vi "AB_1200_1300_Project_Build_Info.vi"(7 "action":T1, 8 "error in (no error)":errorcluster, 10 "buildInfo in":T2, 11 "Object In":T3) -> (0 "error out":errorcluster, 2 "buildInfo out":T2, 3 "Object Out":T3)   [LabVIEW 2020]
uses:
  <vilib>/AppBuilder/RW_Project/AB_RW_Project_PropBag_Action.ctl
  <resource>/Framework/Providers/API/ItemRef.ctl
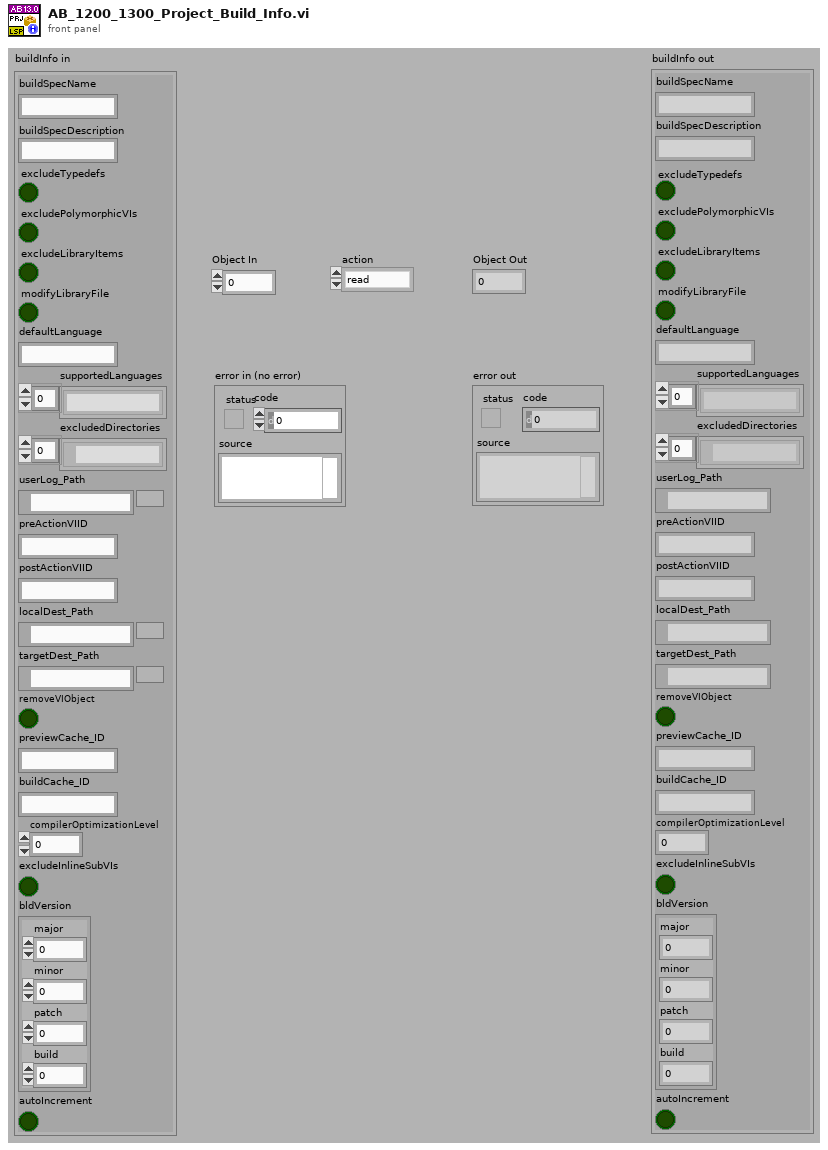
[diagram p1: front panel]
types:
  T1 = typedef "AB_RW_Project_PropBag_Action.ctl" = enum16{"read", "write", "clear", "readPrevious", "writePrevious", "clearPrevious"}
  T2 = cluster{"buildSpecName":string, "buildSpecDescription":string, "excludeTypedefs":bool, "excludePolymorphicVIs":bool, "excludeLibraryItems":bool, "modifyLibraryFile":bool, "defaultLanguage":string, "supportedLanguages":string[], "excludedDirectories":path[], "userLog_Path":path, "preActionVIID":string, "postActionVIID":string, "localDest_Path":path, "targetDest_Path":path, "removeVIObject":bool, "previewCache_ID":string, "buildCache_ID":string, "compilerOptimizationLevel":u32, "excludeInlineSubVIs":bool, "bldVersion":cluster{"major":u16, "minor":u16, "patch":u16, "build":u16}, "autoIncrement":bool}
  T3 = typedef "ItemRef.ctl" = u64
  T4 = cluster{"[0]":i32, "[1]":i32, "[2]":i32, "[3]":i32}
  T5 = cluster{"major":u16, "minor":u16, "patch":u16, "build":u16}
  T6 = typedef "AB_Relative_Path_Type.ctl" = enum16{"<none>", "relativeToCommon", "relativeToAppDir", "relativeToProject"}
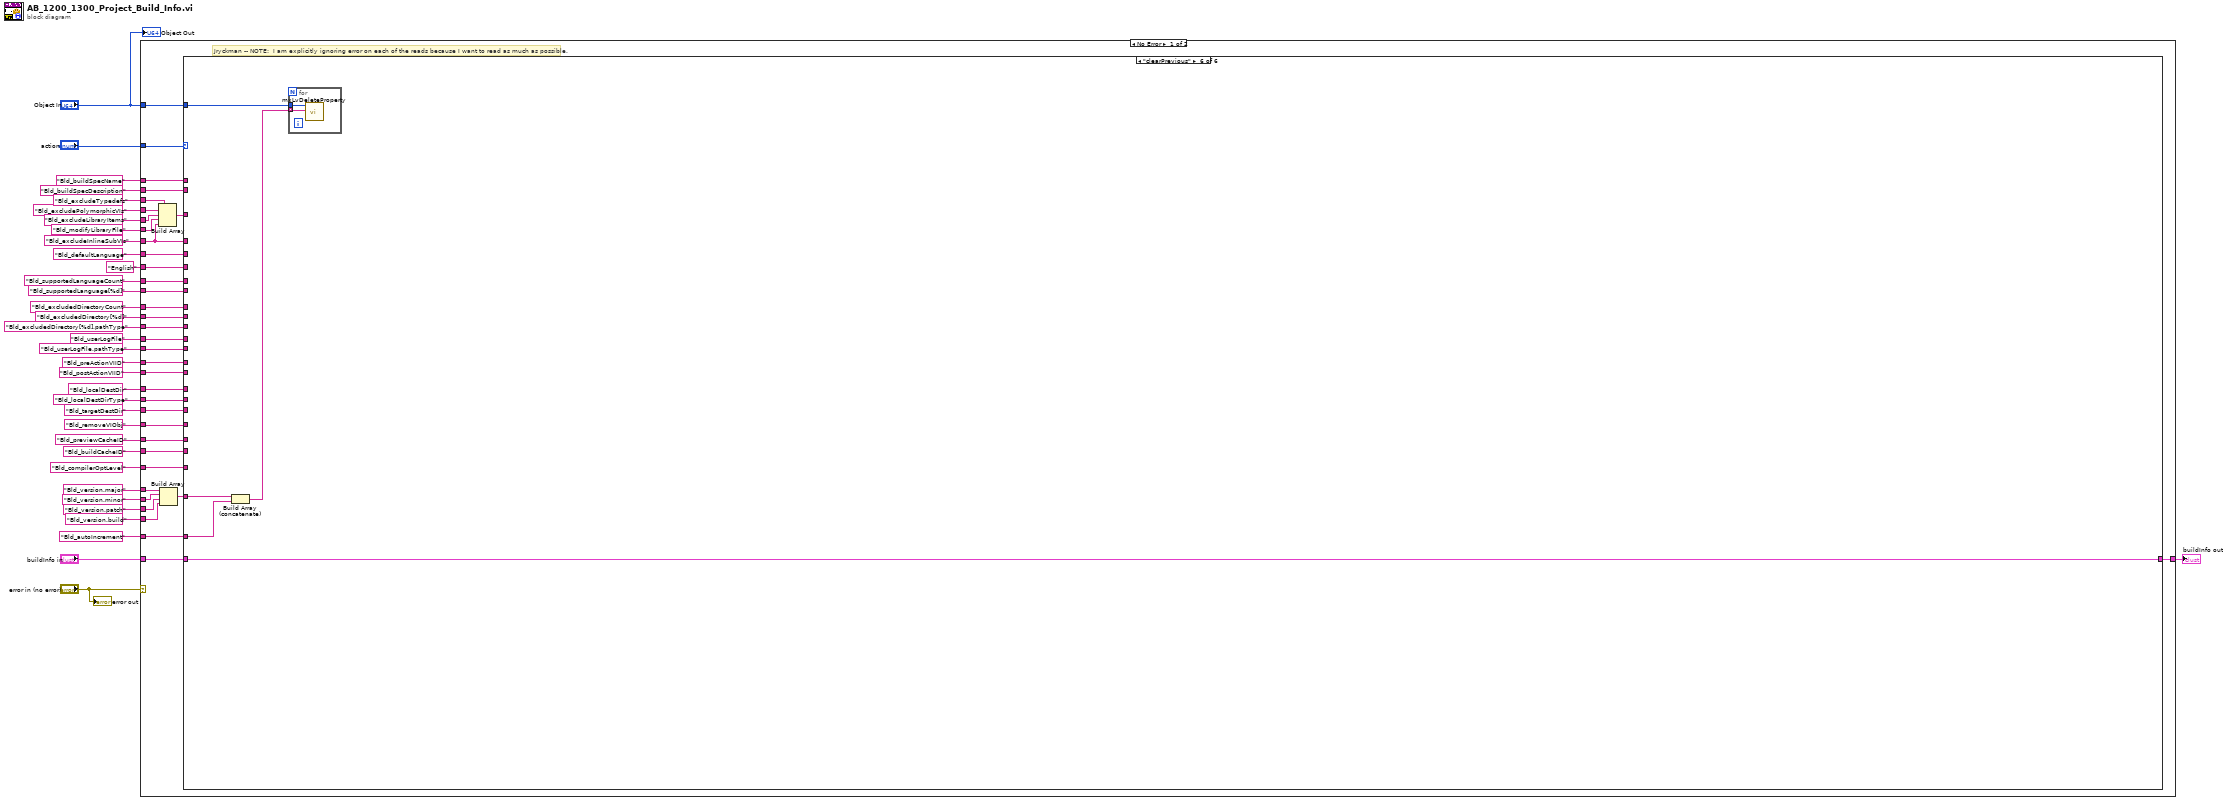
[diagram p0: block diagram]
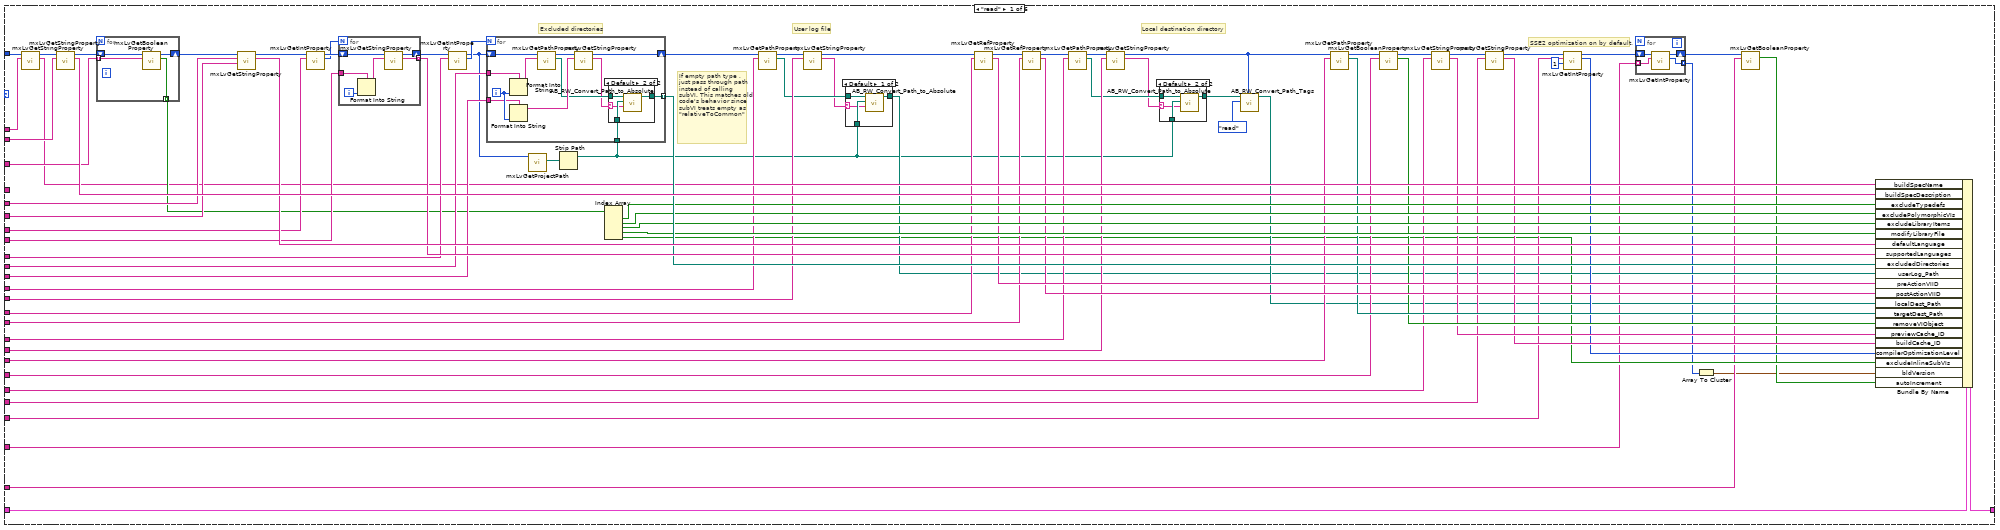
[diagram p2: hidden frame]
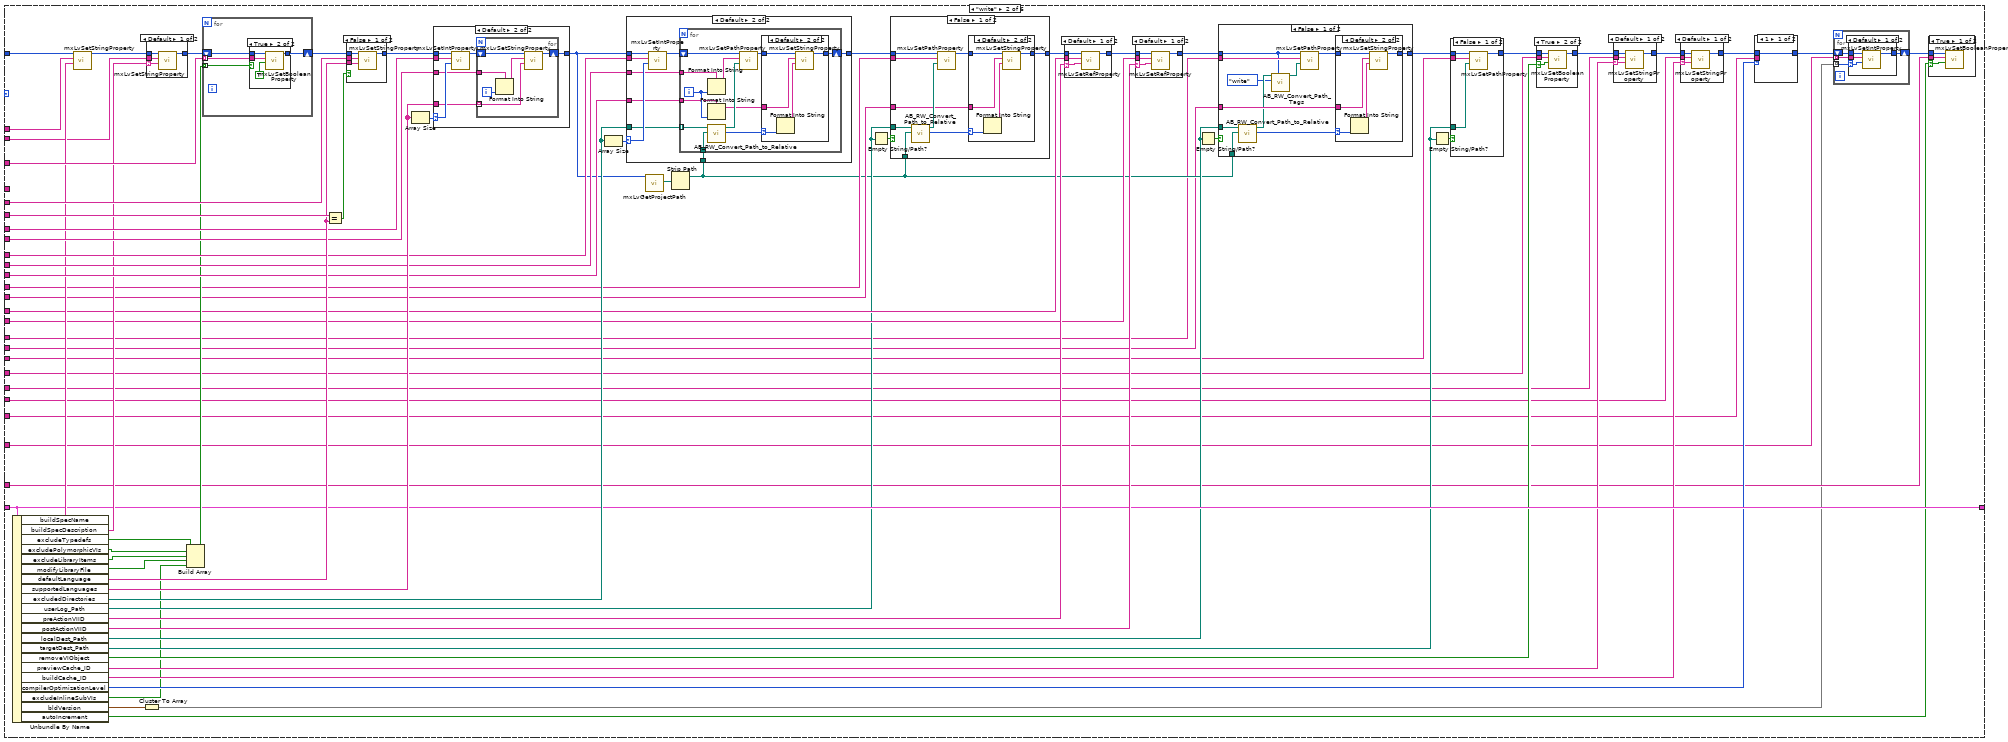
[diagram p6: hidden frame]
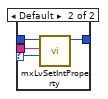
[diagram p9: hidden frame]
diagram:
  n1 = case shown="No Error" "error in (no error)" {
    tunnel: "Object In" -> [w71 _]
    tunnel: [w60 _] -> w33
    tunnel: "Bld_buildSpecDescription" ("Tag") -> [w70 _]
    tunnel: "Bld_excludeTypedefs" ("Tag") -> [w56 _]
    tunnel: "Bld_defaultLanguage" ("Tag") -> [w69 _]
    tunnel: "English" ("Tag") -> [w68 _]
    tunnel: "Bld_supportedLanguageCount" ("Tag") -> [w67 _]
    tunnel: "Bld_supportedLanguage[%d]" ("Tag") -> [w66 _]
    tunnel: "Bld_excludedDirectoryCount" ("Tag") -> [w65 _]
    tunnel: "Bld_excludedDirectory[%d]" ("Tag") -> [w64 _]
    tunnel: "Bld_excludedDirectory[%d].pathType" ("Tag") -> [w63 _]
    tunnel: "buildInfo in" -> [w62 _]
    tunnel: "action" -> [w61 _]
    tunnel: "Bld_excludePolymorphicVIs" ("Tag") -> [w59 _]
    tunnel: "Bld_excludeLibraryItems" ("Tag") -> [w58 _]
    tunnel: "Bld_modifyLibraryFile" ("Tag") -> [w57 _]
    tunnel: "Bld_buildSpecName" ("Tag") -> [w54 _]
    tunnel: "Bld_userLogFile" ("Tag") -> [w53 _]
    tunnel: "Bld_userLogFile.pathType" ("Tag") -> [w52 _]
    tunnel: "Bld_preActionVIID" ("Tag") -> [w51 _]
    tunnel: "Bld_postActionVIID" ("Tag") -> [w50 _]
    tunnel: "Bld_localDestDir" ("Tag") -> [w49 _]
    tunnel: "Bld_targetDestDir" ("Tag") -> [w48 _]
    tunnel: "Bld_localDestDirType" ("Tag") -> [w47 _]
    tunnel: "Bld_removeVIObj" ("Tag") -> [w46 _]
    tunnel: "Bld_previewCacheID" ("Tag") -> [w45 _]
    tunnel: "Bld_buildCacheID" ("Tag") -> [w44 _]
    tunnel: "Bld_compilerOptLevel" ("Tag") -> [w43 _]
    tunnel: "Bld_excludeInlineSubVIs" ("Tag") -> [w42 _]
    tunnel: "Bld_version.major" ("Tag") -> [w40 _]
    tunnel: "Bld_version.minor" ("Tag") -> [w39 _]
    tunnel: "Bld_version.patch" ("Tag") -> [w37 _]
    tunnel: "Bld_version.build" ("Tag") -> [w38 _]
    tunnel: "Bld_autoIncrement" ("Tag") -> [w41 _]
    frame No Error {
      # "Jryckman -- NOTE:  I am explicitly ignoring error on each of the reads because I want to read as much as possible."
      n2 = Build Array(w56, w59, w58, w57, w42) -> (w55:string[])
      n3 = Build Array(w40, w39, w37, w38) -> (w36:string[])
      n4 = case shown="\"clearPrevious\"" w61 {
        tunnel: w71 -> [w124 w243 w448 _ _ w474]
        tunnel: w70 -> [w151 w238 w450 _ _ _]
        tunnel: w69 -> [w149 w263 w449 _ _ _]
        tunnel: w68 -> [w148 w262 _ _ _ _]
        tunnel: w67 -> [w145 w257 w447 _ _ _]
        tunnel: w66 -> [w142 w256 w444 _ _ _]
        tunnel: w65 -> [w139 w252 w440 _ _ _]
        tunnel: w64 -> [w137 w251 w439 _ _ _]
        tunnel: w63 -> [w136 w250 w438 _ _ _]
        tunnel: w62 -> [w133 w222 w435 w470 w471 w476]
        tunnel: [w134 w222 w435 w470 w471 w476] -> w60
        tunnel: w55 -> [w130 w244 w434 _ _ _]
        tunnel: w54 -> [w122 w241 w433 _ _ _]
        tunnel: w53 -> [w117 w235 w431 _ _ _]
        tunnel: w52 -> [w115 w231 w429 _ _ _]
        tunnel: w51 -> [w114 w229 w426 _ _ _]
        tunnel: w50 -> [w111 w226 w425 _ _ _]
        tunnel: w49 -> [w106 w217 w422 _ _ _]
        tunnel: w48 -> [w104 w215 w420 _ _ _]
        tunnel: w47 -> [w105 w218 w421 _ _ _]
        tunnel: w46 -> [w100 w211 w417 _ _ _]
        tunnel: w45 -> [w98 w208 w415 _ _ _]
        tunnel: w44 -> [w95 w205 w413 _ _ _]
        tunnel: w43 -> [w91 w201 w411 _ _ _]
        tunnel: w42 -> [_ _ _ _ _ _]
        tunnel: w41 -> [w74 w196 w407 _ _ w472]
        tunnel: w36 -> [w76 w193 w409 _ _ w473]
        frame "read" {
          # "If empty path type , just pass through path instead of calling subVI. This matches old code's behavior since subVI treats empty as \"relativeToCommon\""
          # "Local destination directory"
          # "User log file"
          # "Excluded directories"
          # "SSE2 optimization on by default."
          n5 = call <resource>:"mxLvGetStringProperty.vi"("Tag"=w122, "Item"=w124) -> ("Value"=w121:string, "Item"=w123:T3)  [unwired: 1 in, 7 out]
          n6 = call <resource>:"mxLvGetStringProperty.vi"("Tag"=w151, "Item"=w123) -> ("Value"=w150:string, "Item"=w132:T3)  [unwired: 1 in, 7 out]
          n7 = for {
            shift-right: [w169] -> w131
            shift-left: w132 -> [w167]
            tunnel: w130 -> [w168] mode=indexing
            tunnel: [w166] -> w129 mode=indexing
            n8 = call <resource>:"mxLvGetBooleanProperty.vi"("Tag"=w168, "Item"=w167) -> ("Value"=w166:bool, "Item"=w169:T3)  [unwired: 1 in, 7 out]
          }
          n9 = call <resource>:"mxLvGetStringProperty.vi"("Default Value (\"\")"=w148, "Tag"=w149, "Item"=w131) -> ("Value"=w147:string, "Item"=w146:T3)  [unwired: 1 in, 6 out]
          n10 = call <resource>:"mxLvGetIntProperty.vi"("Tag"=w145, "Item"=w146) -> ("Value"=w143:i32, "Item"=w144:T3)  [unwired: 1 in, 7 out]
          n11 = for {
            N: w143 -> [_]
            shift-right: [w189] -> w140
            shift-left: w144 -> [w190]
            tunnel: w142 -> [w191]
            tunnel: [w187] -> w141 mode=indexing
            i -> [w192]
            n12 = Format Into String(format string=w191, w192) -> (resulting string=w188:string)  [unwired: 2 in, 1 out]
            n13 = call <resource>:"mxLvGetStringProperty.vi"("Tag"=w188, "Item"=w190) -> ("Value"=w187:string, "Item"=w189:T3)  [unwired: 1 in, 7 out]
          }
          n14 = call <resource>:"mxLvGetIntProperty.vi"("Tag"=w139, "Item"=w140) -> ("Value"=w138:i32, "Item"=w120:T3)  [unwired: 1 in, 7 out]
          n15 = call <resource>:"mxLvGetProjectPath.vi"("Item"=w120) -> ("Project Path"=w119:path)  [unwired: 1 in, 9 out]
          n16 = Strip Path(path=w119) -> (stripped path=w82:path)  [unwired: 1 out]
          n17 = for {
            N: w138 -> [_]
            shift-right: [w174] -> w118
            shift-left: w120 -> [w178]
            tunnel: w137 -> [w181]
            tunnel: w136 -> [w179]
            tunnel: w82 -> [w171]
            tunnel: [w172] -> w135 mode=indexing
            i -> [w180]
            n18 = Format Into String(format string=w181, w180) -> (resulting string=w177:string)  [unwired: 2 in, 1 out]
            n19 = Format Into String(format string=w179, w180) -> (resulting string=w175:string)  [unwired: 2 in, 1 out]
            n20 = call <resource>:"mxLvGetPathProperty.vi"("Tag"=w177, "Item"=w178) -> ("Path"=w173:path, "Item"=w176:T3)  [unwired: 2 in, 6 out]
            n21 = call <resource>:"mxLvGetStringProperty.vi"("Tag"=w175, "Item"=w176) -> ("Value"=w170:string, "Item"=w174:T3)  [unwired: 1 in, 7 out]
            n22 = case shown="Default" w170 {
              selector: w170 -> [_ w183]
              tunnel: w173 -> [w182 w186]
              tunnel: [w182 w185] -> w172
              tunnel: w171 -> [_ w184]
              frame "" {
              }
              frame Default {
                n23 = call <vilib>:"AB_RW_Convert_Path_to_Absolute.vi"("relativeType"=w183, "commonPath"=w184, "relativePath"=w186) -> ("absolute path"=w185:path)  [unwired: 7 in, 1 out]
              }
            }
          }
          n24 = Index Array(array=w129) -> (element #1=w128:bool, element #2=w127:bool, element #3=w126:bool, element #4=w125:bool, element #5=w79:bool)  [unwired: 5 in]
          n25 = call <resource>:"mxLvGetPathProperty.vi"("Tag"=w117, "Item"=w118) -> ("Path"=w86:path, "Item"=w116:T3)  [unwired: 2 in, 6 out]
          n26 = call <resource>:"mxLvGetStringProperty.vi"("Tag"=w115, "Item"=w116) -> ("Value"=w81:string, "Item"=w113:T3)  [unwired: 1 in, 7 out]
          n27 = case shown="Default" w81 {
            selector: w81 -> [w161 _]
            tunnel: w86 -> [w164 w165]
            tunnel: [w163 w165] -> w85
            tunnel: w82 -> [w162 _]
            frame Default {
              n28 = call <vilib>:"AB_RW_Convert_Path_to_Absolute.vi"("relativeType"=w161, "commonPath"=w162, "relativePath"=w164) -> ("absolute path"=w163:path)  [unwired: 7 in, 1 out]
            }
            frame "" {
            }
          }
          n29 = call <resource>:"mxLvGetRefProperty.vi"("Tag"=w114, "Item"=w113) -> ("Value"=w112:string, "Item"=w110:T3)  [unwired: 1 in, 7 out]
          n30 = call <resource>:"mxLvGetRefProperty.vi"("Tag"=w111, "Item"=w110) -> ("Value"=w109:string, "Item"=w107:T3)  [unwired: 1 in, 7 out]
          n31 = call <resource>:"mxLvGetPathProperty.vi"("Tag"=w106, "Item"=w107) -> ("Path"=w84:path, "Item"=w108:T3)  [unwired: 2 in, 6 out]
          n32 = call <resource>:"mxLvGetStringProperty.vi"("Tag"=w105, "Item"=w108) -> ("Value"=w80:string, "Item"=w88:T3)  [unwired: 1 in, 7 out]
          n33 = case shown="Default" w80 {
            selector: w80 -> [_ w157]
            tunnel: w84 -> [w156 w160]
            tunnel: [w156 w159] -> w83
            tunnel: w82 -> [_ w158]
            frame "" {
            }
            frame Default {
              n34 = call <vilib>:"AB_RW_Convert_Path_to_Absolute.vi"("relativeType"=w157, "commonPath"=w158, "relativePath"=w160) -> ("absolute path"=w159:path)  [unwired: 7 in, 1 out]
            }
          }
          n35 = call <vilib>:"AB_RW_Convert_Path_Tags.vi"("buildObject"=w88, "action"=AB_RW_Project_PropBag_Action."read", "Path in"=w83) -> ("Path out"=w89:path)  [unwired: 1 in, 7 out]
          n36 = call <resource>:"mxLvGetPathProperty.vi"("Tag"=w104, "Item"=w88) -> ("Path"=w103:path, "Item"=w102:T3)  [unwired: 2 in, 6 out]
          n37 = call <resource>:"mxLvGetBooleanProperty.vi"("Tag"=w100, "Item"=w102) -> ("Value"=w101:bool, "Item"=w99:T3)  [unwired: 1 in, 7 out]
          n38 = call <resource>:"mxLvGetStringProperty.vi"("Tag"=w98, "Item"=w99) -> ("Value"=w97:string, "Item"=w96:T3)  [unwired: 1 in, 7 out]
          n39 = call <resource>:"mxLvGetStringProperty.vi"("Tag"=w95, "Item"=w96) -> ("Value"=w94:string, "Item"=w93:T3)  [unwired: 1 in, 7 out]
          n40 = call <resource>:"mxLvGetIntProperty.vi"("Default Value (0)"=1, "Tag"=w91, "Item"=w93) -> ("Value"=w92:i32, "Item"=w77:T3)  [unwired: 1 in, 6 out]
          n41 = for {
            shift-right: [w154] -> w75
            shift-left: w77 -> [w155]
            tunnel: w76 -> [w152] mode=indexing
            tunnel: [w153] -> w78 mode=indexing
            n42 = call <resource>:"mxLvGetIntProperty.vi"("Tag"=w152, "Item"=w155) -> ("Value"=w153:i32, "Item"=w154:T3)  [unwired: 1 in, 7 out]
          }
          n43 = Array To Cluster(array=w78) -> (cluster=w72:T4)
          n44 = call <resource>:"mxLvGetBooleanProperty.vi"("Tag"=w74, "Item"=w75) -> ("Value"=w73:bool)  [unwired: 1 in, 8 out]
          n45 = Bundle By Name(cluster=w133, "buildSpecName"=w121, "buildSpecDescription"=w150, "excludeTypedefs"=w128, "excludePolymorphicVIs"=w127, "excludeLibraryItems"=w126, "modifyLibraryFile"=w125, "defaultLanguage"=w147, "supportedLanguages"=w141, "excludedDirectories"=w135, "userLog_Path"=w85, "preActionVIID"=w112, "postActionVIID"=w109, "localDest_Path"=w89, "targetDest_Path"=w103, "removeVIObject"=w101, "previewCache_ID"=w97, "buildCache_ID"=w94, "compilerOptimizationLevel"=w92, "excludeInlineSubVIs"=w79, "bldVersion"=w72, "autoIncrement"=w73) -> (w134:T2)
        }
        frame "write" {
          n46 = Unbundle By Name(w222) -> ("buildSpecName"=w242:string, "buildSpecDescription"=w237:string, "excludeTypedefs"=w249:bool, "excludePolymorphicVIs"=w248:bool, "excludeLibraryItems"=w247:bool, "modifyLibraryFile"=w246:bool, "defaultLanguage"=w261:string, "supportedLanguages"=w255:string[], "excludedDirectories"=w253:path[], "userLog_Path"=w221:path, "preActionVIID"=w228:string, "postActionVIID"=w225:string, "localDest_Path"=w220:path, "targetDest_Path"=w214:path, "removeVIObject"=w210:bool, "previewCache_ID"=w207:string, "buildCache_ID"=w204:string, "compilerOptimizationLevel"=w202:u32, "excludeInlineSubVIs"=w200:bool, "bldVersion"=w195:T5, "autoIncrement"=w197:bool)
          n47 = call <resource>:"mxLvSetStringProperty.vi"("Value (\"\")"=w242, "Tag"=w241, "Item"=w243) -> ("Item"=w240:T3)  [unwired: 2 in, 6 out]
          n48 = Cluster To Array(cluster=w195) -> (array=w194:u16[])
          n49 = case shown="Default" w237 {
            selector: w237 -> [w346 _]
            tunnel: w240 -> [w349 w350]
            tunnel: w238 -> [w348 _]
            tunnel: [w347 w350] -> w239
            frame Default {
              n50 = call <resource>:"mxLvSetStringProperty.vi"("Value (\"\")"=w346, "Tag"=w348, "Item"=w349) -> ("Item"=w347:T3)  [unwired: 2 in, 6 out]
            }
            frame "" {
            }
          }
          n51 = Build Array(w249, w248, w247, w246, w200) -> (w245:bool[])
          n52 = for {
            shift-right: [w353] -> w264
            shift-left: w239 -> [w354]
            tunnel: w245 -> [w352] mode=indexing
            tunnel: w244 -> [w351] mode=indexing
            n53 = case shown="True" w352 {
              tunnel: w354 -> [w355 w359]
              tunnel: [w355 w358] -> w353
              tunnel: w351 -> [_ w357]
              frame False {
              }
              frame True {
                n54 = call <resource>:"mxLvSetBooleanProperty.vi"("Value (F)"=TRUE, "Tag"=w357, "Item"=w359) -> ("Item"=w358:T3)  [unwired: 2 in, 6 out]
              }
            }
          }
          n55 = Equal?(x=w262, y=w261) -> (x = y?=w260:bool)
          n56 = case shown="False" w260 {
            tunnel: w264 -> [w405 w406]
            tunnel: w263 -> [w404 _]
            tunnel: w261 -> [w403 _]
            tunnel: [w402 w406] -> w258
            frame False {
              n57 = call <resource>:"mxLvSetStringProperty.vi"("Value (\"\")"=w403, "Tag"=w404, "Item"=w405) -> ("Item"=w402:T3)  [unwired: 2 in, 6 out]
            }
            frame True {
            }
          }
          n58 = Array Size(array=w255) -> (size(s)=w259:i32)
          n59 = case shown="Default" w259 {
            selector: w259 -> [_ w393]
            tunnel: w258 -> [w388 w395]
            tunnel: w257 -> [_ w394]
            tunnel: w256 -> [_ w391]
            tunnel: w255 -> [_ w390]
            tunnel: [w388 w389] -> w232
            frame 0 {
            }
            frame Default {
              n60 = call <resource>:"mxLvSetIntProperty.vi"("Value (0)"=w393, "Tag"=w394, "Item"=w395) -> ("Item"=w392:T3)  [unwired: 2 in, 6 out]
              n61 = for {
                shift-right: [w400] -> w389
                shift-left: w392 -> [w401]
                tunnel: w391 -> [w398]
                tunnel: w390 -> [w396] mode=indexing
                i -> [w399]
                n62 = Format Into String(format string=w398, w399) -> (resulting string=w397:string)  [unwired: 2 in, 1 out]
                n63 = call <resource>:"mxLvSetStringProperty.vi"("Value (\"\")"=w396, "Tag"=w397, "Item"=w401) -> ("Item"=w400:T3)  [unwired: 2 in, 6 out]
              }
            }
          }
          n64 = Array Size(array=w253) -> (size(s)=w254:i32)
          n65 = call <resource>:"mxLvGetProjectPath.vi"("Item"=w232) -> ("Project Path"=w233:path)  [unwired: 1 in, 9 out]
          n66 = Strip Path(path=w233) -> (stripped path=w219:path)  [unwired: 1 out]
          n67 = case shown="Default" w254 {
            selector: w254 -> [_ w368]
            tunnel: w232 -> [w360 w363]
            tunnel: w252 -> [_ w369]
            tunnel: w251 -> [_ w366]
            tunnel: w253 -> [_ w365]
            tunnel: w250 -> [_ w364]
            tunnel: [w360 w362] -> w236
            tunnel: w219 -> [_ w361]
            frame 0 {
            }
            frame Default {
              n68 = call <resource>:"mxLvSetIntProperty.vi"("Value (0)"=w368, "Tag"=w369, "Item"=w363) -> ("Item"=w367:T3)  [unwired: 2 in, 6 out]
              n69 = for {
                shift-right: [w381] -> w362
                shift-left: w367 -> [w377]
                tunnel: w366 -> [w380]
                tunnel: w365 -> [w379] mode=indexing
                tunnel: w361 -> [w371]
                tunnel: w364 -> [w370]
                i -> [w375]
                n70 = Format Into String(format string=w380, w375) -> (resulting string=w378:string)  [unwired: 2 in, 1 out]
                n71 = Format Into String(format string=w370, w375) -> (resulting string=w373:string)  [unwired: 2 in, 1 out]
                n72 = call <vilib>:"AB_RW_Convert_Path_to_Relative.vi"("commonPath"=w371, "absolutePath"=w379) -> ("relativeType"=w372:T6, "newPath"=w374:path)  [unwired: 1 in, 7 out]
                n73 = call <resource>:"mxLvSetPathProperty.vi"("Path"=w374, "Tag"=w378, "Item"=w377) -> ("Item"=w376:T3)  [unwired: 2 in, 6 out]
                n74 = case shown="Default" w372 {
                  selector: w372 -> [_ w383]
                  tunnel: [w382 w387] -> w381
                  tunnel: w376 -> [w382 w386]
                  tunnel: w373 -> [_ w384]
                  frame "<none>" {
                  }
                  frame Default {
                    n75 = Format Into String(w383) -> (resulting string=w385:string)  [unwired: 3 in, 1 out]
                    n76 = call <resource>:"mxLvSetStringProperty.vi"("Value (\"\")"=w385, "Tag"=w384, "Item"=w386) -> ("Item"=w387:T3)  [unwired: 2 in, 6 out]
                  }
                }
              }
            }
          }
          n77 = Empty String/Path?(string/path=w221) -> (empty?=w234:bool)
          n78 = case shown="False" w234 {
            tunnel: w236 -> [w338 w345]
            tunnel: w235 -> [w337 _]
            tunnel: w219 -> [w334 _]
            tunnel: w221 -> [w333 _]
            tunnel: w231 -> [w331 _]
            tunnel: [w330 w345] -> w230
            frame False {
              n79 = call <vilib>:"AB_RW_Convert_Path_to_Relative.vi"("commonPath"=w334, "absolutePath"=w333) -> ("relativeType"=w336:T6, "newPath"=w332:path)  [unwired: 1 in, 7 out]
              n80 = call <resource>:"mxLvSetPathProperty.vi"("Path"=w332, "Tag"=w337, "Item"=w338) -> ("Item"=w335:T3)  [unwired: 2 in, 6 out]
              n81 = case shown="Default" w336 {
                selector: w336 -> [_ w341]
                tunnel: w335 -> [w339 w344]
                tunnel: w331 -> [_ w342]
                tunnel: [w339 w340] -> w330
                frame "<none>" {
                }
                frame Default {
                  n82 = Format Into String(w341) -> (resulting string=w343:string)  [unwired: 3 in, 1 out]
                  n83 = call <resource>:"mxLvSetStringProperty.vi"("Value (\"\")"=w343, "Tag"=w342, "Item"=w344) -> ("Item"=w340:T3)  [unwired: 2 in, 6 out]
                }
              }
            }
            frame True {
            }
          }
          n84 = case shown="Default" w228 {
            selector: w228 -> [w326 _]
            tunnel: w230 -> [w328 w329]
            tunnel: w229 -> [w327 _]
            tunnel: [w325 w329] -> w227
            frame Default {
              n85 = call <resource>:"mxLvSetRefProperty.vi"("Value (\"\")"=w326, "Tag"=w327, "Item"=w328) -> ("Item"=w325:T3)  [unwired: 2 in, 6 out]
            }
            frame "" {
            }
          }
          n86 = case shown="Default" w225 {
            selector: w225 -> [w321 _]
            tunnel: w227 -> [w323 w324]
            tunnel: w226 -> [w322 _]
            tunnel: [w320 w324] -> w223
            frame Default {
              n87 = call <resource>:"mxLvSetRefProperty.vi"("Value (\"\")"=w321, "Tag"=w322, "Item"=w323) -> ("Item"=w320:T3)  [unwired: 2 in, 6 out]
            }
            frame "" {
            }
          }
          n88 = Empty String/Path?(string/path=w220) -> (empty?=w224:bool)
          n89 = case shown="False" w224 {
            tunnel: w223 -> [w302 w319]
            tunnel: w217 -> [w312 _]
            tunnel: w219 -> [w309 _]
            tunnel: w220 -> [w308 _]
            tunnel: w218 -> [w307 _]
            tunnel: [w306 w319] -> w216
            frame False {
              n90 = call <vilib>:"AB_RW_Convert_Path_to_Relative.vi"("commonPath"=w309, "absolutePath"=w308) -> ("relativeType"=w311:T6, "newPath"=w305:path)  [unwired: 1 in, 7 out]
              n91 = call <vilib>:"AB_RW_Convert_Path_Tags.vi"("buildObject"=w302, "action"=AB_RW_Project_PropBag_Action."write", "Path in"=w305) -> ("Path out"=w304:path)  [unwired: 1 in, 7 out]
              n92 = call <resource>:"mxLvSetPathProperty.vi"("Path"=w304, "Tag"=w312, "Item"=w302) -> ("Item"=w310:T3)  [unwired: 2 in, 6 out]
              n93 = case shown="Default" w311 {
                selector: w311 -> [_ w315]
                tunnel: w310 -> [w313 w318]
                tunnel: w307 -> [_ w316]
                tunnel: [w313 w314] -> w306
                frame "<none>" {
                }
                frame Default {
                  n94 = Format Into String(w315) -> (resulting string=w317:string)  [unwired: 3 in, 1 out]
                  n95 = call <resource>:"mxLvSetStringProperty.vi"("Value (\"\")"=w317, "Tag"=w316, "Item"=w318) -> ("Item"=w314:T3)  [unwired: 2 in, 6 out]
                }
              }
            }
            frame True {
            }
          }
          n96 = Empty String/Path?(string/path=w214) -> (empty?=w213:bool)
          n97 = case shown="False" w213 {
            tunnel: w216 -> [w300 w301]
            tunnel: w215 -> [w299 _]
            tunnel: w214 -> [w298 _]
            tunnel: [w297 w301] -> w212
            frame False {
              n98 = call <resource>:"mxLvSetPathProperty.vi"("Path"=w298, "Tag"=w299, "Item"=w300) -> ("Item"=w297:T3)  [unwired: 2 in, 6 out]
            }
            frame True {
            }
          }
          n99 = case shown="True" w210 {
            selector: w210 -> [_ w294]
            tunnel: w212 -> [w292 w296]
            tunnel: w211 -> [_ w295]
            tunnel: [w292 w293] -> w209
            frame False {
            }
            frame True {
              n100 = call <resource>:"mxLvSetBooleanProperty.vi"("Value (F)"=w294, "Tag"=w295, "Item"=w296) -> ("Item"=w293:T3)  [unwired: 2 in, 6 out]
            }
          }
          n101 = case shown="Default" w207 {
            selector: w207 -> [w288 _]
            tunnel: w209 -> [w290 w291]
            tunnel: w208 -> [w289 _]
            tunnel: [w287 w291] -> w206
            frame Default {
              n102 = call <resource>:"mxLvSetStringProperty.vi"("Value (\"\")"=w288, "Tag"=w289, "Item"=w290) -> ("Item"=w287:T3)  [unwired: 2 in, 6 out]
            }
            frame "" {
            }
          }
          n103 = case shown="Default" w204 {
            selector: w204 -> [w283 _]
            tunnel: w206 -> [w285 w286]
            tunnel: w205 -> [w284 _]
            tunnel: [w282 w286] -> w203
            frame Default {
              n104 = call <resource>:"mxLvSetStringProperty.vi"("Value (\"\")"=w283, "Tag"=w284, "Item"=w285) -> ("Item"=w282:T3)  [unwired: 2 in, 6 out]
            }
            frame "" {
            }
          }
          n105 = case shown="1" w202 {
            selector: w202 -> [_ w280]
            tunnel: w203 -> [w277 w281]
            tunnel: w201 -> [_ w279]
            tunnel: [w277 w278] -> w199
            frame 1 {
            }
            frame Default {
              n106 = call <resource>:"mxLvSetIntProperty.vi"("Value (0)"=w280, "Tag"=w279, "Item"=w281) -> ("Item"=w278:T3)  [unwired: 2 in, 6 out]
            }
          }
          n107 = for {
            tunnel: w194 -> [w270] mode=indexing
            shift-right: [w269] -> w198
            shift-left: w199 -> [w271]
            tunnel: w193 -> [w268] mode=indexing
            n108 = case shown="Default" w270 {
              selector: w270 -> [w274 _]
              tunnel: w271 -> [w275 w276]
              tunnel: w268 -> [w273 _]
              tunnel: [w272 w276] -> w269
              frame Default {
                n109 = call <resource>:"mxLvSetIntProperty.vi"("Value (0)"=w274, "Tag"=w273, "Item"=w275) -> ("Item"=w272:T3)  [unwired: 2 in, 6 out]
              }
              frame 0 {
              }
            }
          }
          n110 = case shown="True" w197 {
            selector: w197 -> [w266 _]
            tunnel: w198 -> [w267 _]
            tunnel: w196 -> [w265 _]
            frame True {
              n111 = call <resource>:"mxLvSetBooleanProperty.vi"("Value (F)"=w266, "Tag"=w265, "Item"=w267) -> ()  [unwired: 2 in, 7 out]
            }
            frame False {
            }
          }
        }
        frame "clear" {
          n112 = Build Array (concatenate)(w433, w450, w434, w449, w447, w440) -> (w436:string[])
          n113 = call <resource>:"mxLvGetIntProperty.vi"("Tag"=w447, "Item"=w448) -> ("Value"=w445:i32, "Item"=w446:T3)  [unwired: 1 in, 7 out]
          n114 = for {
            N: w445 -> [_]
            shift-right: [w466] -> w441
            shift-left: w446 -> [w467]
            tunnel: w444 -> [w468]
            i -> [w469]
            n115 = Format Into String(format string=w468, w469) -> (resulting string=w465:string)  [unwired: 2 in, 1 out]
            n116 = call <resource>:"mxLvDeleteProperty.vi"("Tag"=w465, "Item"=w467) -> ("Item"=w466:T3)  [unwired: 1 in, 8 out]
          }
          n117 = call <resource>:"mxLvGetIntProperty.vi"("Tag"=w440, "Item"=w441) -> ("Value"=w443:i32, "Item"=w442:T3)  [unwired: 1 in, 7 out]
          n118 = for {
            N: w443 -> [_]
            shift-right: [w460] -> w437
            shift-left: w442 -> [w463]
            tunnel: w439 -> [w464]
            tunnel: w438 -> [w458]
            i -> [w459]
            n119 = Format Into String(format string=w464, w459) -> (resulting string=w462:string)  [unwired: 2 in, 1 out]
            n120 = Format Into String(format string=w458, w459) -> (resulting string=w457:string)  [unwired: 2 in, 1 out]
            n121 = call <resource>:"mxLvDeleteProperty.vi"("Tag"=w462, "Item"=w463) -> ("Item"=w461:T3)  [unwired: 1 in, 8 out]
            n122 = call <resource>:"mxLvDeleteProperty.vi"("Tag"=w457, "Item"=w461) -> ("Item"=w460:T3)  [unwired: 1 in, 8 out]
          }
          n123 = for {
            tunnel: w436 -> [w455] mode=indexing
            shift-right: [w454] -> w432
            shift-left: w437 -> [w456]
            n124 = call <resource>:"mxLvDeleteProperty.vi"("Tag"=w455, "Item"=w456) -> ("Item"=w454:T3)  [unwired: 1 in, 8 out]
          }
          n125 = call <resource>:"mxLvDeleteProperty.vi"("Tag"=w431, "Item"=w432) -> ("Item"=w430:T3)  [unwired: 1 in, 8 out]
          n126 = call <resource>:"mxLvDeleteProperty.vi"("Tag"=w429, "Item"=w430) -> ("Item"=w427:T3)  [unwired: 1 in, 8 out]
          n127 = call <resource>:"mxLvDeleteProperty.vi"("Tag"=w426, "Item"=w427) -> ("Item"=w428:T3)  [unwired: 1 in, 8 out]
          n128 = call <resource>:"mxLvDeleteProperty.vi"("Tag"=w425, "Item"=w428) -> ("Item"=w419:T3)  [unwired: 1 in, 8 out]
          n129 = call <resource>:"mxLvDeleteProperty.vi"("Tag"=w422, "Item"=w419) -> ("Item"=w424:T3)  [unwired: 1 in, 8 out]
          n130 = call <resource>:"mxLvDeleteProperty.vi"("Tag"=w421, "Item"=w424) -> ("Item"=w423:T3)  [unwired: 1 in, 8 out]
          n131 = call <resource>:"mxLvDeleteProperty.vi"("Tag"=w420, "Item"=w423) -> ("Item"=w418:T3)  [unwired: 1 in, 8 out]
          n132 = call <resource>:"mxLvDeleteProperty.vi"("Tag"=w417, "Item"=w418) -> ("Item"=w416:T3)  [unwired: 1 in, 8 out]
          n133 = call <resource>:"mxLvDeleteProperty.vi"("Tag"=w415, "Item"=w416) -> ("Item"=w414:T3)  [unwired: 1 in, 8 out]
          n134 = call <resource>:"mxLvDeleteProperty.vi"("Tag"=w413, "Item"=w414) -> ("Item"=w412:T3)  [unwired: 1 in, 8 out]
          n135 = call <resource>:"mxLvDeleteProperty.vi"("Tag"=w411, "Item"=w412) -> ("Item"=w410:T3)  [unwired: 1 in, 8 out]
          n136 = for {
            tunnel: w409 -> [w452] mode=indexing
            shift-right: [w451] -> w408
            shift-left: w410 -> [w453]
            n137 = call <resource>:"mxLvDeleteProperty.vi"("Tag"=w452, "Item"=w453) -> ("Item"=w451:T3)  [unwired: 1 in, 8 out]
          }
          n138 = call <resource>:"mxLvDeleteProperty.vi"("Tag"=w407, "Item"=w408) -> ()  [unwired: 1 in, 9 out]
        }
        frame "readPrevious" {
        }
        frame "writePrevious" {
        }
        frame "clearPrevious" {
          n139 = Build Array (concatenate)(w473, w472) -> (w475:string[])
          n140 = for {
            tunnel: w474 -> [w478]
            tunnel: w475 -> [w477] mode=indexing
            n141 = call <resource>:"mxLvDeleteProperty.vi"("Tag"=w477, "Item"=w478) -> ()  [unwired: 1 in, 9 out]
          }
        }
      }
    }
    frame Error {
    }
  }
  "buildInfo out" <- w33
  "Object Out" <- "Object In"
  "error out" <- "error in (no error)"
